vi "TextWithValue.vi"(4 "precision":i16=2, 5 "IsError":bool, 6 "[User-specified Font].Size":i16=18, 7 "Visible":bool=TRUE, 8 "Origin":cluster{"X":i32, "Y":i32}, 9 "Value":dbl=5500.0, 10 "Header":string="RPM: ", 11 "Refnum in":T1=refnum) -> (3 "Refnum out":T1)   [LabVIEW 2015]
uses:
  <vilib>/vision/Image Controls.llb/IMAQ Image.ctl
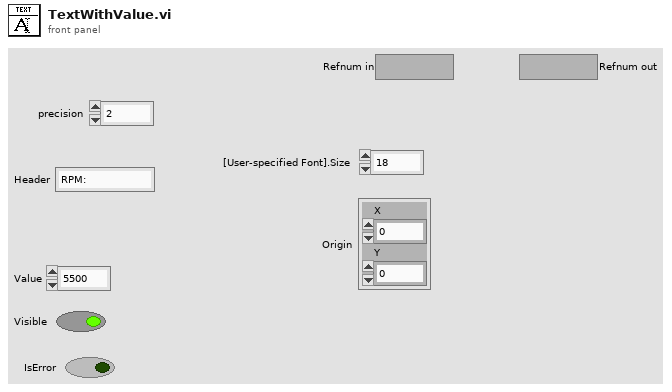
[diagram p1: front panel]
types:
  T1 = typedef "IMAQ Image.ctl" = refnum<image>
  T2 = cluster{"Desired Font (Application)":enum16{"User-specified Font", "Application Font", "System Font", "Dialog Font"}, "[User-specified Font]":cluster{"Font Name":string, "Size":i16, "Strikeout?":bool, "Italic?":bool, "Underline?":bool, "Outline?":bool, "Shadow?":bool, "Bold?":bool, "Rotation Angle":dbl}, "Horizontal Alignment":i16, "Vertical Alignment":i16}
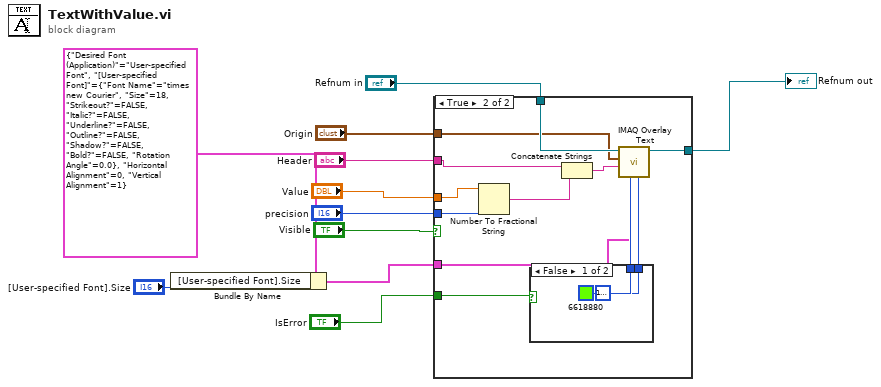
[diagram p0: block diagram]
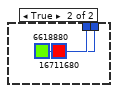
[diagram p3: hidden frame]
diagram:
  n1 = Bundle By Name(cluster=T2 {"Desired Font (Application)"=enum."User-specified Font", "[User-specified Font]"={"Font Name"="times new Courier", "Size"=18, "Strikeout?"=FALSE, "Italic?"=FALSE, "Underline?"=FALSE, "Outline?"=FALSE, "Shadow?"=FALSE, "Bold?"=FALSE, "Rotation Angle"=0.0}, "Horizontal Alignment"=0, "Vertical Alignment"=1} ("Font, Size & Style"), "[User-specified Font].Size"="[User-specified Font].Size") -> (w1:T2)
  n2 = case shown="True" "Visible" {
    tunnel: "Refnum in" -> [w12 w24]
    tunnel: [w12 w23] -> w9
    tunnel: "IsError" -> [_ w19]
    tunnel: "Origin" -> [_ w18]
    tunnel: "Value" -> [_ w16]
    tunnel: "Header" -> [_ w17]
    tunnel: "precision" -> [_ w14]
    tunnel: w1 -> [_ w13]
    frame False {
    }
    frame True {
      n3 = Number To Fractional String(number=w16, precision (6)=w14) -> (F-format string=w15:string)  [unwired: 2 in]
      n4 = case shown="False" w19 {
        tunnel: [u32 6618880 ("Text Color (black)") u32 6618880 ("Text Color (black)")] -> w21
        tunnel: [u32 16777216 ("BG Color (Transparent)") u32 16711680 ("BG Color (Transparent)")] -> w20
        frame False {
        }
        frame True {
        }
      }
      n5 = Concatenate Strings(w17, w15) -> (w22:string)
      n6 = call "IMAQ Overlay Text"("BG Color (Transparent)"=w20, "Text Color (black)"=w21, "Font, Size & Style"=w13, "String"=w22, "Origin"=w18, "Image"=w24) -> ("Image Out"=w23:T1)  [unwired: 4 in, 1 out]
    }
  }
  "Refnum out" <- w9
